vi "Post-Build Action.vi"(5 "Files Generated by Build":path[](array[path]), 6 "Top Level/Always Included VIs":path[](array[path]), 7 "Destination Path":path, 8 "error in (no error)":errorcluster, 9 "Target Name":string, 10 "Build Specification Name":string, 11 "Project Path":path) -> (0 "error out":errorcluster)   [LabVIEW 2018]
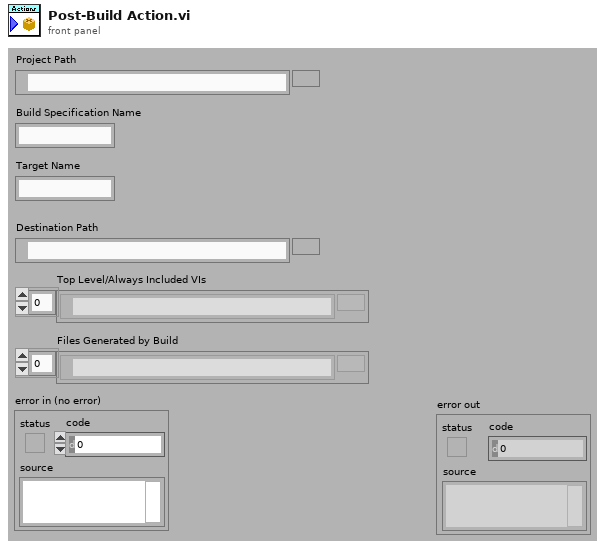
[diagram p1: front panel]
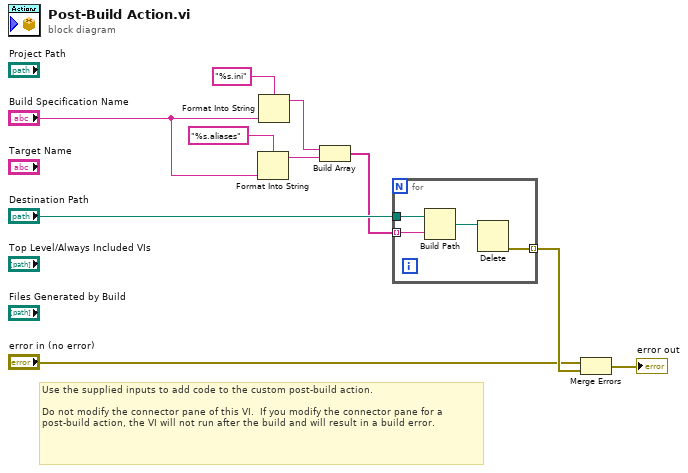
[diagram p0: block diagram]
diagram:
  # "Use the supplied inputs to add code to the custom post-build action.\n\nDo not modify the connector pane of this VI.  If you modify the connector pane for a post-build action, the VI will not run after the build and will result in a build error."
  n1 = Format Into String(format string="%s.aliases", "Build Specification Name") -> (resulting string=w5:string)  [unwired: 2 in, 1 out]
  n2 = Format Into String(format string="%s.ini", "Build Specification Name") -> (resulting string=w6:string)  [unwired: 2 in, 1 out]
  n3 = Build Array(w6, w5) -> (w4:string[])
  n4 = for {
    tunnel: "Destination Path" -> [w14]
    tunnel: w4 -> [w13] mode=indexing
    tunnel: [w11] -> w3 mode=indexing
    n5 = Build Path(base path=w14, name or relative path=w13) -> (appended path=w12:path)
    n6 = Delete(path (use dialog)=w12) -> (error out=w11:errorcluster)  [unwired: 4 in, 2 out]
  }
  n7 = Merge Errors("error in (no error)", w3) -> (→"error out":errorcluster)
